vi "Add Report Information.vi"(8 "error in (no error)":errorcluster, 10 "Report Information.lvclass":refnum<class "Report Information.lvclass">, 11 "ResultProcessor in":refnum<class "ResultProcessor.lvclass">) -> (0 "error out":errorcluster, 3 "ResultProcessor out":refnum<class "ResultProcessor.lvclass">)   [LabVIEW 2015, in "ResultProcessor.lvclass"]
doc: "This VI adds an entire set of Report Information. This will overwrite any of the previously written Report Information elements."
uses:
  ResultProcessor.lvclass
  Report Information/Report Information.lvclass
  CommandQueueDataType.ctl
  Result/Result.lvclass
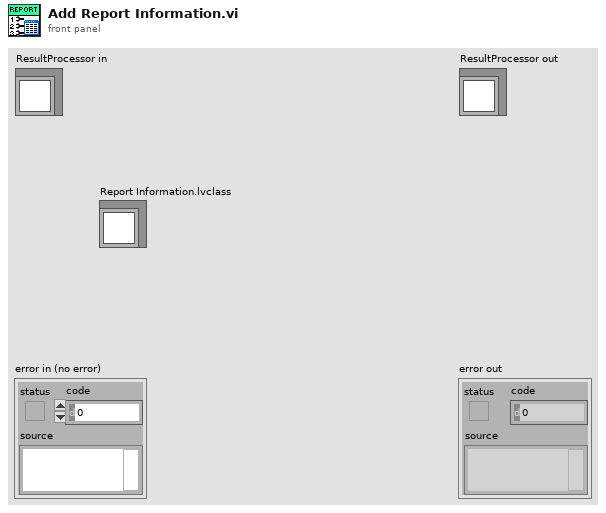
[diagram p1: front panel]
types:
  T1 = typedef "ResultProcessor.lvclass/CommandQueueDataType.ctl" = cluster{"Command":enum16{"New Report", "Add Result", "Publish Report", "Shutdown", "Add DUT Information", "Add Station Information", "Add Report Information", "Add Test Information"}, "Report Information.lvclass":refnum<class "Report Information.lvclass">, "Result.lvclass":refnum<class "Result.lvclass">}
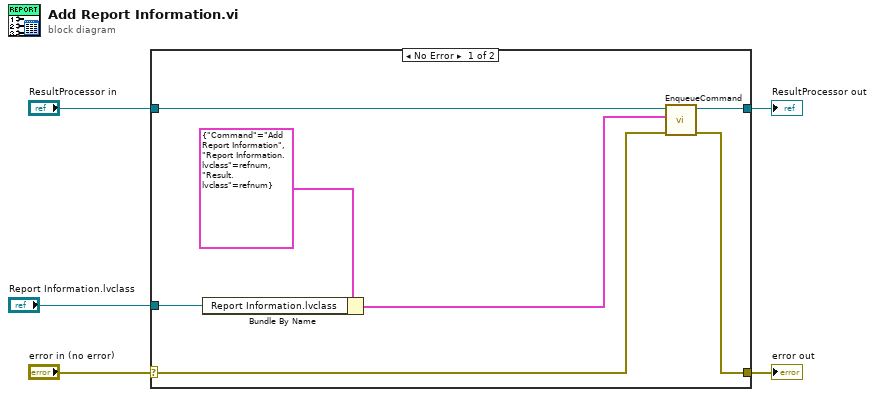
[diagram p0: block diagram]
diagram:
  n1 = case shown="No Error" "error in (no error)" {
    selector: "error in (no error)" -> [w10 w14]
    tunnel: [w9 w14] -> w4
    tunnel: [w11 w13] -> w2
    tunnel: "ResultProcessor in" -> [w12 w13]
    tunnel: "Report Information.lvclass" -> [w6 _]
    frame No Error {
      n2 = Bundle By Name(cluster=T1 {"Command"=enum."Add Report Information", "Report Information.lvclass"=refnum, "Result.lvclass"=refnum} ("element"), "Report Information.lvclass"=w6) -> (w7:T1)
      n3 = call "EnqueueCommand.vi"("error in (no error)"=w10, "element"=w7, "ResultProcessor in"=w12) -> ("error out"=w9:errorcluster, "ResultProcessor out"=w11:refnum<class "ResultProcessor.lvclass">)  [unwired: 7 in]
    }
    frame Error {
    }
  }
  "error out" <- w4
  "ResultProcessor out" <- w2
